vi "setOutBits.vi"(9 "outBit2":bool, 10 "outBit1":bool, 11 "outBit0":bool) -> ()   [LabVIEW 2014]
uses:
  <vilib>/rvi/eio/common/nirviEmuTemplateMethod_errors.vi
  <vilib>/eio/EIONode/EIONode.xnode
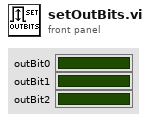
[diagram p1: front panel]
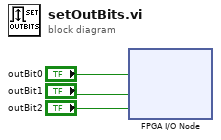
[diagram p0: block diagram]
diagram:
  n1 = xnode "FPGA I/O Node"("OutBit0"="outBit0", "OutBit1"="outBit1", "OutBit2"="outBit2") -> ()  [unwired: 3 in, 3 out]
